vi "PixieCalcCountData.vi"(9 "PixieTimes":T1, 10 "Histogram Data":u32[][](array[numeric]), 11 "CrsrList":T3) -> (2 "Count Data":T2)   [LabVIEW 2013]
uses:
  <vilib>/Utility/miscctls.llb/LVCursorListTypeDef.ctl
  ctl/PixieTimes.ctl
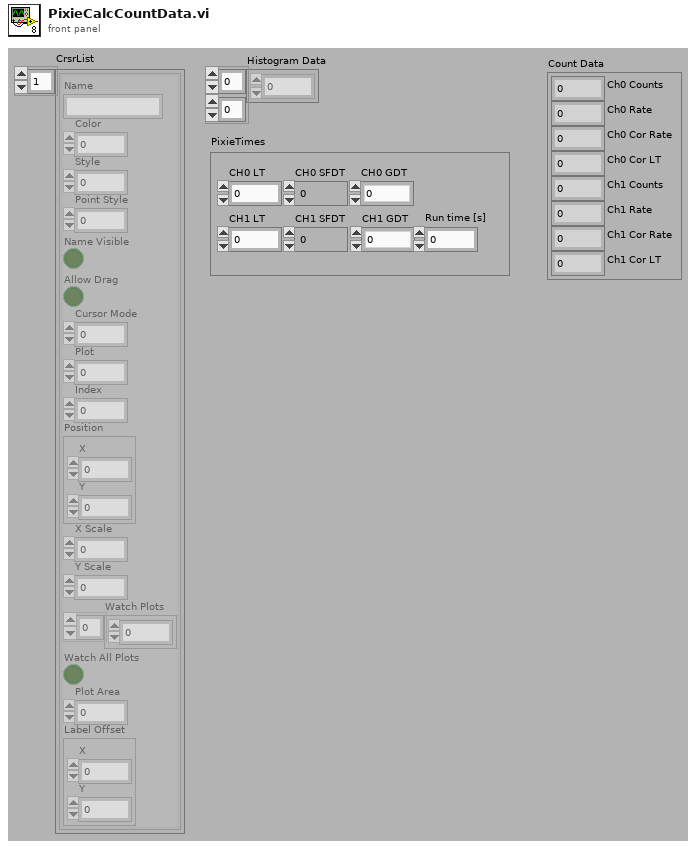
[diagram p1: front panel]
types:
  T1 = typedef "PixieTimes.ctl" = cluster{"CH0 LT":dbl, "CH1 LT":dbl, "CH0 SFDT":dbl, "CH1 SFDT":dbl, "CH0 GDT":dbl, "CH1 GDT":dbl, "Run time [s]":dbl}
  T2 = cluster{"Ch0 Counts":u32, "Ch0 Rate":dbl, "Ch0 Cor Rate":dbl, "Ch0 Cor LT":dbl, "Ch1 Counts":u32, "Ch1 Rate":dbl, "Ch1 Cor Rate":dbl, "Ch1 Cor LT":dbl}
  T3 = typedef "LVCursorListTypeDef.ctl" = cluster{"Name":string, "Color":u32, "Style":u8, "Point Style":u8, "Name Visible":bool, "Allow Drag":bool, "Cursor Mode":u32, "Plot":i32, "Index":i32, "Position":cluster{"X":dbl, "Y":dbl}, "X Scale":u32, "Y Scale":u32, "Watch Plots":i32[], "Watch All Plots":bool, "Plot Area":i32, "Label Offset":cluster{"X":dbl, "Y":dbl}}[]
  T4 = cluster{"Name":string, "Color":u32, "Style":u8, "Point Style":u8, "Name Visible":bool, "Allow Drag":bool, "Cursor Mode":u32, "Plot":i32, "Index":i32, "Position":cluster{"X":dbl, "Y":dbl}, "X Scale":u32, "Y Scale":u32, "Watch Plots":i32[], "Watch All Plots":bool, "Plot Area":i32, "Label Offset":cluster{"X":dbl, "Y":dbl}}
  T5 = cluster{"Ch0 Counts":u32, "Rate":dbl, "Cor Rate":dbl, "Cor LT":dbl, "Ch1 Counts":u32, "Rate":dbl, "Cor Rate":dbl, "Cor LT":dbl}
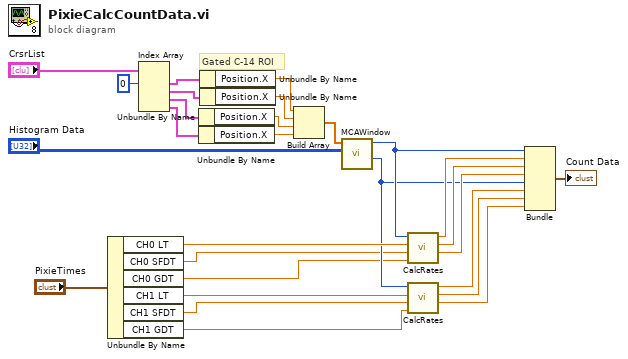
[diagram p0: block diagram]
diagram:
  # "Gated C-14 ROI"
  n1 = Unbundle By Name("PixieTimes") -> ("CH0 LT"=w15:dbl, "CH0 SFDT"=w5:dbl, "CH0 GDT"=w4:dbl, "CH1 LT"=w3:dbl, "CH1 SFDT"=w2:dbl, "CH1 GDT"=w1:dbl)
  n2 = Index Array(array="CrsrList", index #1=0 ("index")) -> (element #1=w25:T4, element #2=w26:T4, element #3=w27:T4, element #4=w28:T4)  [unwired: 3 in]
  n3 = Unbundle By Name(w27) -> ("Position.X"=w18:dbl)
  n4 = Unbundle By Name(w28) -> ("Position.X"=w20:dbl)
  n5 = Unbundle By Name(w25) -> ("Position.X"=w22:dbl)
  n6 = Unbundle By Name(w26) -> ("Position.X"=w21:dbl)
  n7 = Build Array(w22, w21, w18, w20) -> (w19:dbl[])
  n8 = call "MCAWindow.vi"("Histogram Data"="Histogram Data", "Window"=w19) -> ("Ch1 Counts"=w7:u32, "Ch0 Counts"=w14:u32)  [unwired: 4 in, 4 out]
  n9 = call "CalcRates.vi"("GDT"=w4, "SFDT"=w5, "LT"=w15, "Counts"=w14) -> ("Cor LT"=w11:dbl, "Cor Rate"=w12:dbl, "Rate"=w13:dbl)  [unwired: 5 in]
  n10 = call "CalcRates.vi"("GDT"=w1, "SFDT"=w2, "LT"=w3, "Counts"=w7) -> ("Cor LT"=w8:dbl, "Cor Rate"=w9:dbl, "Rate"=w10:dbl)  [unwired: 5 in]
  n11 = Bundle("Ch0 Counts"=w14, "Rate"=w13, "Cor Rate"=w12, "Cor LT"=w11, "Ch1 Counts"=w7, "Rate"=w10, "Cor Rate"=w9, "Cor LT"=w8) -> (→"Count Data":T5)  [unwired: 1 in]
